vi "configuration UI.vi"() -> ()   [LabVIEW 2013, in "TEC editor node.lvclass"]
uses:
  TEC editor node.lvclass
  <vilib>/CEF_TreeControl/Node/NodeRef.ctl
  <vilib>/CEF_TreeControl/Node/NISE_CEF_Node.lvclass
  <vilib>/NI/AMC/Message Queue.ctl
  <vilib>/NI/AMC/Message.ctl
  <vilib>/NI/Tools/Keyed Array/KeyedArray.ctl
  <vilib>/CEF_TreeControl/Node/UserEventRef.ctl
  <vilib>/CEF_TreeControl/Controls/EventCluster.ctl
  <vilib>/NI/Tag Bus Data Framework/Configuration Editor/Classes/Engine Parent/Engine Parent Editor Node.lvclass
  <vilib>/NI/Tag Bus/tag/tag descriptor.lvclass
  <vilib>/NI/Tag Bus/tag/Data Type.ctl
  module/configuration/TEC configuration.lvclass
  <vilib>/NI/Module Execution Interface/Engine Configuration/engine configuration.lvclass
  <vilib>/NI/Tag Bus/tag/tag descriptor.lvclass/tag descriptor.ctl
  TEC editor node.lvclass/TEC editor node.ctl
  <vilib>/NI/Tag Bus Module Framework/channel/channel classification.ctl
  <vilib>/NI/Tag Bus Module Framework/root configuration/TBM configuration.lvclass/TBM configuration.ctl
  <vilib>/NI/Tag Bus/tag/write tag name.vi
  <vilib>/NI/Tag Bus/tag/write data type.vi
  <vilib>/NI/Tag Bus Module Framework/root configuration/create GUID.vi
  <vilib>/NI/Tag Bus Data Framework/Configuration Editor/Classes/Module editor node/module editor node.lvclass
  <vilib>/CEF_TreeControl/NISE_CEF_TreeControl.lvlib
  <vilib>/NI/Tag Bus Module Framework/channel/TBM channel.lvclass
  <vilib>/NI/Tag Bus Module Framework/root configuration/TBM configuration.lvclass
  <vilib>/NI/Tools/Keyed Array/Tools_KeyedArray.lvlib
  <vilib>/NI/AMC/AMC.lvlib
panel:
  in  "Tab Control":enum32{"Channel Mapping"}(tab)
  in  "Direction":T1(radio)
  in  "remove to":bool
  in  "add to":bool
  in  "remove from":bool
  in  "add from":bool
  in  "toCVTlist":i32(listbox)
  in  "fromCVTlist":i32(listbox)
  in  "avail tags":i32(listbox)=-1
  in  "user event":T2
  in  "main queue":T3
  in  "node ref":T4
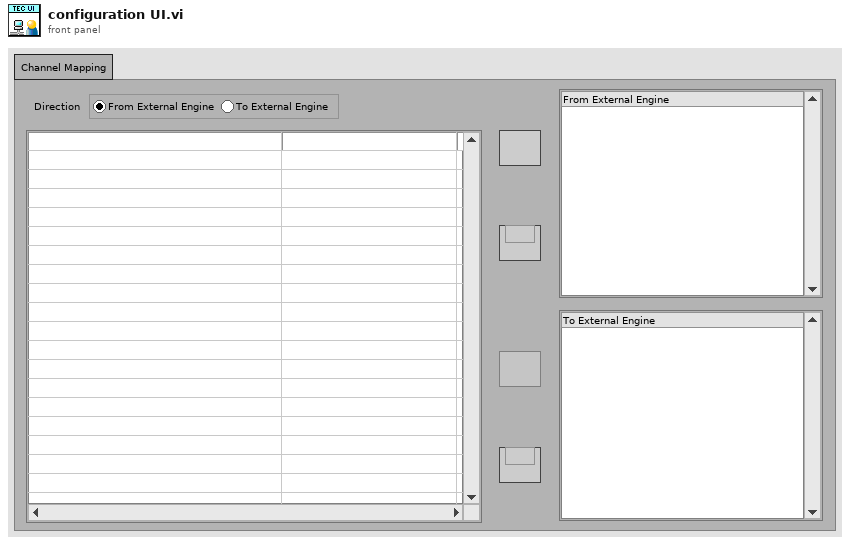
[diagram p1: front panel]
types:
  T1 = enum32{"From External Engine", "To External Engine"}
  T2 = typedef "NISE_CEF_Node.lvclass/UserEventRef.ctl" = refnum<user-event>
  T3 = typedef "AMC.lvlib/Message Queue.ctl" = refnum<queue>
  T4 = typedef "NISE_CEF_Node.lvclass/NodeRef.ctl" = refnum<data-value>
  T5 = typedef "NISE_CEF_TreeControl.lvlib/EventCluster.ctl" = cluster{"command":string, "data":string}
  T6 = typedef "tag bus.lvlib/tag descriptor.lvclass/Data Type.ctl" = enum16{"Double", "Single", "I64", "I32", "I16", "I8", "U64", "U32", "U16", "U8", "Boolean", "String", "Array of Double", "Array of Single", "Array of I64", "Array of I32", "Array of I16", "Array of I8", "Array of U64", "Array of U32", "Array of U16", "Array of U8", "Array of Boolean", "Array of String"}
  T7 = enum8{"Enabled", "Disabled", "Disabled and Grayed Out"}
  T8 = typedef "TBM channel.lvclass/channel classification.ctl" = enum16{"input data", "output data", "processing parameter", "processing result"}
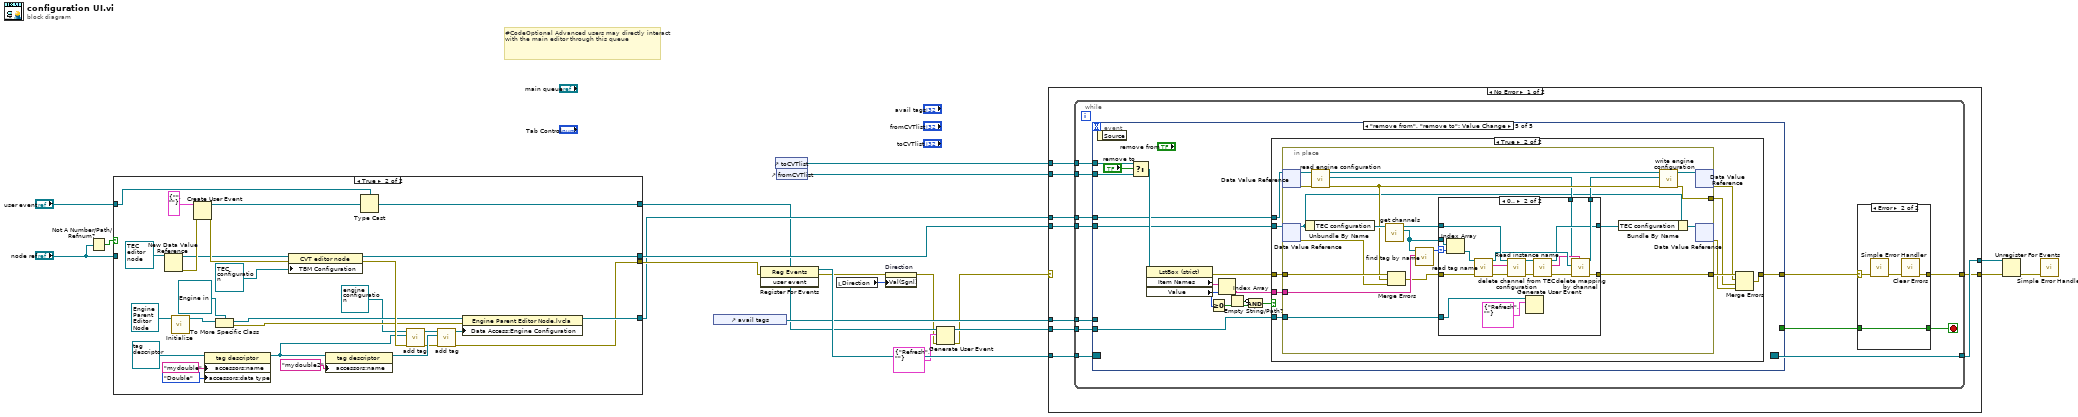
[diagram p0: block diagram]
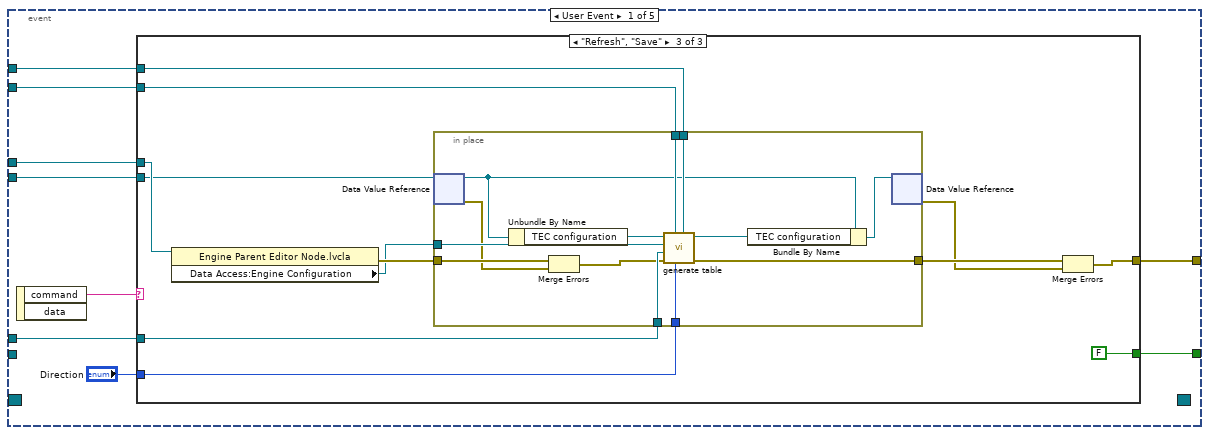
[diagram p3: hidden frame]
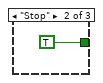
[diagram p5: hidden frame]
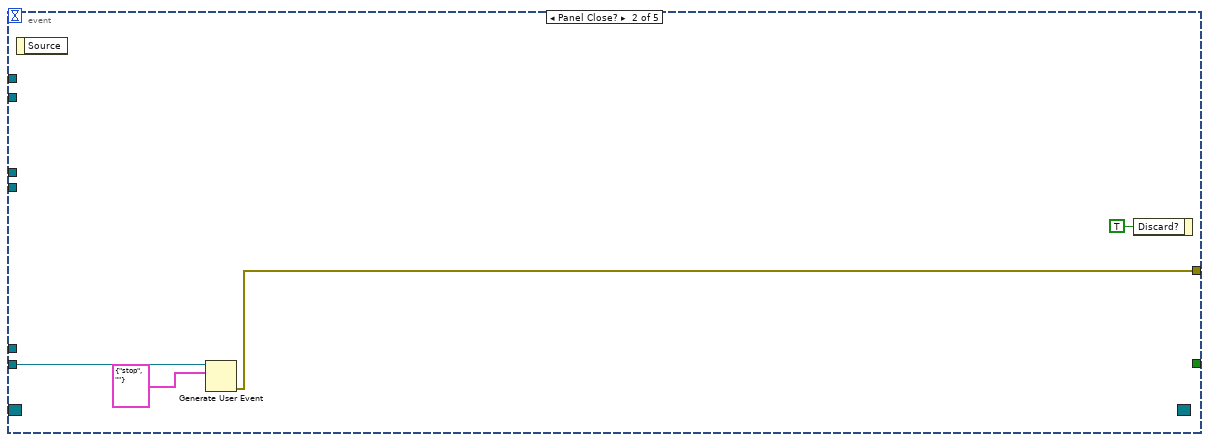
[diagram p6: hidden frame]
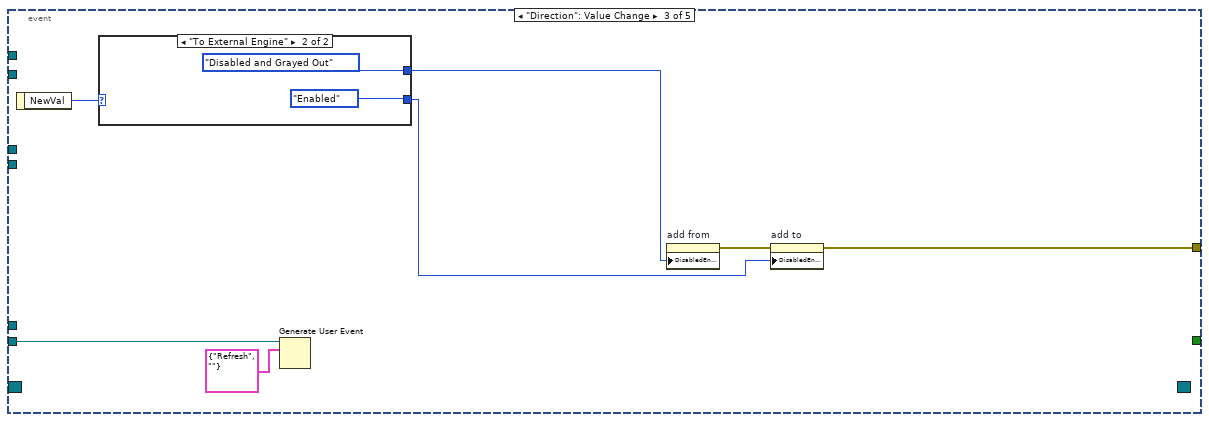
[diagram p7: hidden frame]
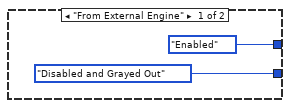
[diagram p8: hidden frame]
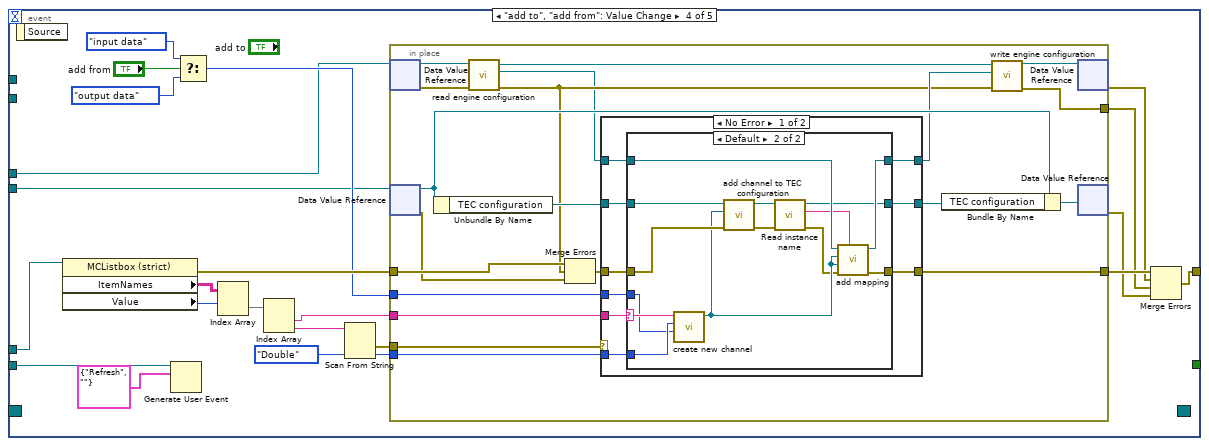
[diagram p9: hidden frame]
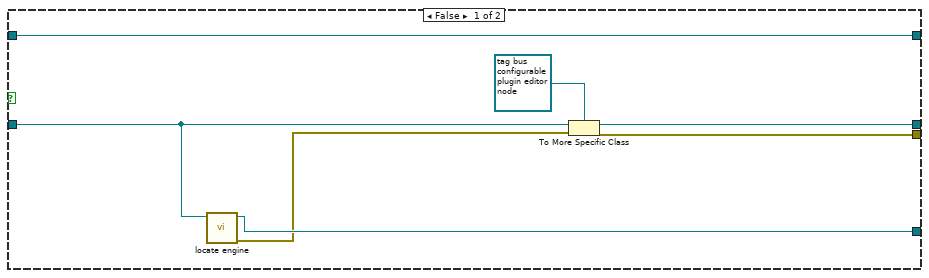
[diagram p15: hidden frame]
diagram:
  # "#CodeOptional Advanced users may directly interact with the main editor through this queue"
  n1 = Not A Number/Path/Refnum?(number/path/refnum="node ref") -> (NaN/Path/Refnum?=w17:bool)
  n2 = case shown="True" w17 {
    tunnel: "user event" -> [w27 w32]
    tunnel: [w27 w33] -> w3
    tunnel: "node ref" -> [w25 _]
    tunnel: [w24 w51] -> w14
    tunnel: [w23 w42] -> w13
    tunnel: [w22 w48] -> w11
    frame False {
      n3 = call <vilib>:"locate engine.vi"("component"=w25) -> ("error out"=w21:errorcluster, "engine"=w22:refnum<data-value>)  [unwired: 9 in]
      n4 = To More Specific Class(target class=refnum<data-value> refnum ("data value reference"), reference=w25, error in=w21) -> (specific class reference=w24:refnum<data-value>, error out=w23:errorcluster)
    }
    frame True {
      n5 = New Data Value Reference(data value=refnum<class "TEC editor node.lvclass"> refnum ("tag bus configurable plugin editor node")) -> (data value reference=w50:refnum<data-value>, error out=w53:errorcluster)  [unwired: 1 in]
      n6 = call-dynamic "Initialize.vi"("Engine in"=refnum<class "Engine Parent Editor Node.lvclass"> refnum) -> ("data value reference"=w37:T4)  [unwired: 8 in, 2 out]
      n7 = Create User Event(user event datatype=T5 {"command"="", "data"=""} ("event data"), error in=w53) -> (user event=w54:refnum<user-event>, error out=w52:errorcluster)
      n8 = property class="tag descriptor"(reference=refnum<class "tag descriptor.lvclass"> refnum ("tag descriptor"), "accessors:name"="mydouble" ("name"), "accessors:data type"=Data_Type."Double" ("data type")) -> (reference out=w40:refnum<class "tag descriptor.lvclass">)  [unwired: 1 in, 1 out]
      n9 = To More Specific Class(target class=refnum<data-value> refnum ("data value reference"), reference=w37) -> (specific class reference=w36:refnum<data-value>, error out=w34:errorcluster)  [unwired: 1 in]
      n10 = property class="CVT editor node"(reference=w50, error in=w52, "TBM Configuration"=refnum<class "TEC configuration.lvclass"> refnum ("CVT configuration")) -> (reference out=w51:refnum<data-value>, error out=w44:errorcluster)
      n11 = property class="tag descriptor"(reference=w40, "accessors:name"="mydouble2" ("name")) -> (reference out=w41:refnum<class "tag descriptor.lvclass">)  [unwired: 1 in, 1 out]
      n12 = Type Cast(type=w32, x=w54) -> (*(type *) &x=w33:T2)
      n13 = call <vilib>:"add tag.vi"("error in"=w44, "tag descriptor"=w40, "engine configuration in"=refnum<class "engine configuration.lvclass"> refnum) -> ("error out"=w31:errorcluster, "engine configuration out"=w30:refnum<class "engine configuration.lvclass">)  [unwired: 7 in]
      n14 = call <vilib>:"add tag.vi"("error in"=w31, "tag descriptor"=w41, "engine configuration in"=w30) -> ("error out"=w42:errorcluster, "engine configuration out"=w29:refnum<class "engine configuration.lvclass">)  [unwired: 7 in]
      n15 = property class="Engine Parent Editor Node.lvcla"(reference=w36, error in=w34, "Data Access:Engine Configuration"=w29) -> (reference out=w48:refnum<data-value>)  [unwired: 1 out]
    }
  }
  n16 = control-ref of="avail tags"() -> (w10:refnum<vi>)
  n17 = register-events(error in=w13, w3) -> (reference out=w20:refnum<event-registration>, error out=w7:errorcluster)  [unwired: 1 in]
  n18 = control-ref of="toCVTlist"() -> (w9:refnum<vi>)
  n19 = control-ref of="fromCVTlist"() -> (w8:refnum<vi>)
  n20 = local read "Direction"() -> (w6:T1)
  n21 = property on="Direction" class="RadioBtnsControl (strict)"(error in=w7, "Val(Sgnl)"=w6) -> (error out=w2:errorcluster)  [unwired: 1 in, 1 out]
  n22 = Generate User Event(user event=w3, event data cluster=T5 {"command"="Refresh", "data"=""} ("event data"), error in=w2) -> (user event out=w4:T2, error out=w1:errorcluster)  [unwired: 1 in]
  n23 = case shown="No Error" w1 {
    selector: w1 -> [_ w274]
    tunnel: w20 -> [w64 w273]
    tunnel: [w63 w273] -> w19
    tunnel: [w62 w274] -> w18
    tunnel: w14 -> [w61 _]
    tunnel: w11 -> [w60 _]
    tunnel: w10 -> [w59 _]
    tunnel: w9 -> [w58 _]
    tunnel: w8 -> [w57 _]
    tunnel: w4 -> [w56 _]
    frame No Error {
      n24 = while {
        tunnel: w64 -> [w76]
        tunnel: [w75] -> w63
        tunnel: w61 -> [w70]
        tunnel: w60 -> [w69]
        tunnel: w56 -> [w68]
        tunnel: w59 -> [w67]
        tunnel: w58 -> [w66]
        tunnel: w57 -> [w65]
        tunnel: [w71] -> w62
        stop <- w73 stop-if-true
        n25 = event shown="[4] \"remove from\", \"remove to\": Value Change" {
          selector: w76 -> [_ _ _ _ _]
          dyn-events: [_ _ _ _ _] -> w75
          timeout: _ -> [_ _ _ _ _]
          tunnel: [w91 _ _ _ _] -> w72
          tunnel: [w89 w118 w125 w138 w209] -> w74
          tunnel: w70 -> [w88 _ _ w134 w206]
          tunnel: w69 -> [w87 _ _ w135 w205]
          tunnel: w68 -> [_ w119 w127 w154 w208]
          tunnel: w67 -> [w86 _ _ w148 _]
          tunnel: w66 -> [w85 _ _ _ w218]
          tunnel: w65 -> [w84 _ _ _ w219]
          event User Event {
            n26 = event-data() -> ("command"=w90:string)  [unwired: 1 in, 1 out]
            n27 = case shown="\"Refresh\", \"Save\"" w90 {
              tunnel: [_ TRUE FALSE] -> w91
              tunnel: [_ _ w94] -> w89
              tunnel: w88 -> [_ _ w95]
              tunnel: w87 -> [_ _ w97]
              tunnel: w86 -> [_ _ w102]
              tunnel: w85 -> [_ _ w101]
              tunnel: w84 -> [_ _ w100]
              tunnel: "Direction" -> [_ _ w99]
              frame Default {
              }
              frame "Stop" {
              }
              frame "Refresh", "Save" {
                n28 = property class="Engine Parent Editor Node.lvcla"(reference=w97) -> (error out=w98:errorcluster, "Data Access:Engine Configuration"=w96:refnum<class "engine configuration.lvclass">)  [unwired: 1 in, 1 out]
                n29 = in-place {
                  in-place-border: [w117] -> w103
                  in-place-border: w102 -> [w116]
                  in-place-border: w101 -> [w115]
                  in-place-border: w100 -> [w114]
                  in-place-border: w99 -> [w113]
                  in-place-border: w98 -> [w112]
                  in-place-border: w96 -> [w111]
                  n30 = in-place-dvr #1(w95) -> (w107:refnum<class "TEC editor node.lvclass">, w109:errorcluster)
                  n31 = Unbundle By Name(w107) -> ("TEC configuration"=w108:refnum<class "TEC configuration.lvclass">)
                  n32 = Merge Errors(w112, w109) -> (w110:errorcluster)
                  n33 = call "generate table.vi"("to TEC"=w115, "Direction"=w113, "from TEC"=w114, "error in"=w110, "avail tags"=w116, "engine configuration in"=w111, "TEC in"=w108) -> ("error out"=w117:errorcluster, "TEC out"=w105:refnum<class "TEC configuration.lvclass">)  [unwired: 3 in]
                  n34 = Bundle By Name(cluster=w107, "TEC configuration"=w105) -> (w106:refnum<class "TEC editor node.lvclass">)
                  n35 = in-place-dvr #1(w106) -> (w93:errorcluster)  [unwired: 1 out]
                }
                n36 = Merge Errors(w103, w93) -> (w94:errorcluster)
              }
            }
          }
          event Panel Close? {
            n37 = event-data() -> ()  [unwired: 1 in, 1 out]
            n38 = Generate User Event(user event=w119, event data cluster=T5 {"command"="stop", "data"=""} ("event data")) -> (error out=w118:errorcluster)  [unwired: 2 in, 1 out]
            n39 = event-data("Discard?"=TRUE) -> ()  [unwired: 1 in, 1 out]
          }
          event "Direction": Value Change {
            n40 = event-data() -> ("NewVal"=w124:T1)  [unwired: 1 in]
            n41 = case shown="\"To External Engine\"" w124 {
              tunnel: [T7."Enabled" ("Disabled") T7."Disabled and Grayed Out" ("Disabled")] -> w123
              tunnel: [T7."Disabled and Grayed Out" ("Disabled") T7."Enabled" ("Disabled")] -> w122
              frame "From External Engine" {
              }
              frame "To External Engine" {
              }
            }
            n42 = Generate User Event(user event=w127, event data cluster=T5 {"command"="Refresh", "data"=""} ("event data")) -> ()  [unwired: 2 in, 2 out]
            n43 = property on="add from" class="Bool"("DisabledEnum"=w123) -> (error out=w126:errorcluster)  [unwired: 2 in, 1 out]
            n44 = property on="add to" class="Bool"(error in=w126, "DisabledEnum"=w122) -> (error out=w125:errorcluster)  [unwired: 1 in, 1 out]
          }
          event "add to", "add from": Value Change {
            n45 = event-data() -> ()  [unwired: 1 in, 1 out]
            n46 = property class="MCListbox (strict)"(reference=w148) -> (error out=w149:errorcluster, "ItemNames"=w147:string[][], "Value"=w146:i32)  [unwired: 1 in, 1 out]
            n47 = Generate User Event(user event=w154, event data cluster=T5 {"command"="Refresh", "data"=""} ("event data")) -> ()  [unwired: 2 in, 2 out]
            n48 = Select(t=channel_classification."input data" ("channel classification"), s="add from", f=channel_classification."output data" ("channel classification")) -> (s? t:f=w139:T8)
            n49 = Index Array(array=w147, index (row)=w146) -> (element=w143:string[])  [unwired: 1 in]
            n50 = Index Array(array=w143) -> (element #1=w142:string, element #2=w145:string)  [unwired: 2 in]
            n51 = Scan From String(input string=w145, default 1=Data_Type."Double" ("data type")) -> (error out=w141:errorcluster, output 1=w140:T6)  [unwired: 3 in, 2 out]
            n52 = in-place {
              in-place-border: [w175] -> w155
              in-place-border: w149 -> [w174]
              in-place-border: w142 -> [w173]
              in-place-border: w141 -> [w172]
              in-place-border: w140 -> [w171]
              in-place-border: w139 -> [w170]
              in-place-border: [w160] -> w133
              n53 = in-place-dvr #2(w135) -> (w163:refnum<class "Engine Parent Editor Node.lvclass">, w158:errorcluster)
              n54 = in-place-dvr #3(w134) -> (w166:refnum<class "TEC editor node.lvclass">, w164:errorcluster)
              n55 = Unbundle By Name(w166) -> ("TEC configuration"=w168:refnum<class "TEC configuration.lvclass">)
              n56 = call <vilib>:"read engine configuration.vi"("error in"=w158, "Engine Parent Editor Node in"=w163) -> ("error out"=w157:errorcluster, "engine configuration"=w156:refnum<class "engine configuration.lvclass">, "Engine Parent Editor Node out"=w159:refnum<class "Engine Parent Editor Node.lvclass">)  [unwired: 7 in]
              n57 = Merge Errors(w174, w157, w164) -> (w169:errorcluster)
              n58 = case shown="No Error" w172 {
                tunnel: [w184 w202] -> w175
                tunnel: [w183 w204] -> w161
                tunnel: [w182 w203] -> w167
                tunnel: w168 -> [w181 w203]
                tunnel: w156 -> [w180 w204]
                tunnel: w169 -> [w179 w202]
                tunnel: w173 -> [w178 _]
                tunnel: w171 -> [w177 _]
                tunnel: w170 -> [w176 _]
                frame No Error {
                  n59 = case shown="Default" w178 {
                    selector: w178 -> [_ w195]
                    tunnel: [w187 w201] -> w184
                    tunnel: w179 -> [w187 w197]
                    tunnel: w180 -> [w185 w200]
                    tunnel: [w186 w189] -> w182
                    tunnel: w181 -> [w186 w198]
                    tunnel: [w185 w199] -> w183
                    tunnel: w177 -> [_ w194]
                    tunnel: w176 -> [_ w193]
                    frame "" {
                    }
                    frame Default {
                      n60 = call <vilib>:"create new channel.vi"("channel classification"=w193, "data type"=w194, "channel name"=w195) -> ("channel"=w192:refnum<class "TBM channel.lvclass">)  [unwired: 8 in]
                      n61 = call "add channel to TEC configuration.vi"("error in"=w197, "channel"=w192, "TEC configuration in"=w198) -> ("error out"=w196:errorcluster, "TEC configuration out"=w190:refnum<class "TEC configuration.lvclass">)  [unwired: 7 in]
                      n62 = call <vilib>:"Read instance name.vi"("error in"=w196, "configuration in"=w190) -> ("error out"=w191:errorcluster, "instance id"=w188:string, "configuration out"=w189:refnum<class "TEC configuration.lvclass">)  [unwired: 7 in]
                      n63 = call <vilib>:"add mapping.vi"("owner ID"=w188, "error in"=w191, "channel"=w192, "tag descriptor"=w192, "engine configuration"=w200) -> ("error out"=w201:errorcluster, "engine configuration out"=w199:refnum<class "engine configuration.lvclass">)  [unwired: 5 in]
                    }
                  }
                }
                frame Error {
                }
              }
              n64 = Bundle By Name(cluster=w166, "TEC configuration"=w167) -> (w165:refnum<class "TEC editor node.lvclass">)
              n65 = call <vilib>:"write engine configuration.vi"("error in"=w157, "engine configuration"=w161, "Engine Parent Editor Node in"=w159) -> ("error out"=w160:errorcluster, "Engine Parent Editor Node out"=w162:refnum<class "Engine Parent Editor Node.lvclass">)  [unwired: 7 in]
              n66 = in-place-dvr #2(w162) -> (w137:errorcluster)  [unwired: 1 out]
              n67 = in-place-dvr #3(w165) -> (w136:errorcluster)  [unwired: 1 out]
            }
            n68 = Merge Errors(w155, w137, w133, w136) -> (w138:errorcluster)
          }
          event "remove from", "remove to": Value Change {
            n69 = event-data() -> ()  [unwired: 1 in, 1 out]
            n70 = Select(t=w218, s="remove to", f=w219) -> (s? t:f=w216:refnum<vi>)
            n71 = property class="LstBox (strict)"(reference=w216) -> (error out=w210:errorcluster, "Item Names"=w215:string[], "Value"=w214:i32)  [unwired: 1 in, 1 out]
            n72 = Greater Or Equal To 0?(x=w214) -> (x >= 0?=w212:bool)
            n73 = Index Array(array=w215, index=w214) -> (element=w207:string)
            n74 = Empty String/Path?(string/path=w207) -> (empty?=w213:bool)
            n75 = Compound Arithmetic op=AND(invert w213, w212) -> (w211:bool)
            n76 = case shown="True" w211 {
              tunnel: w210 -> [w220 w227]
              tunnel: [w220 w226] -> w209
              tunnel: w208 -> [_ w230]
              tunnel: w207 -> [_ w229]
              tunnel: w206 -> [_ w225]
              tunnel: w205 -> [_ w224]
              frame False {
              }
              frame True {
                n77 = in-place {
                  in-place-border: w230 -> [w251]
                  in-place-border: w229 -> [w250]
                  in-place-border: [w247] -> w228
                  in-place-border: w227 -> [w246]
                  in-place-border: [w240] -> w221
                  n78 = in-place-dvr #4(w224) -> (w243:refnum<class "Engine Parent Editor Node.lvclass">, w238:errorcluster)
                  n79 = in-place-dvr #5(w225) -> (w233:refnum<class "TEC editor node.lvclass">, w237:errorcluster)
                  n80 = Unbundle By Name(w233) -> ("TEC configuration"=w239:refnum<class "TEC configuration.lvclass">)
                  n81 = call <vilib>:"read engine configuration.vi"("error in"=w238, "Engine Parent Editor Node in"=w243) -> ("error out"=w236:errorcluster, "engine configuration"=w235:refnum<class "engine configuration.lvclass">, "Engine Parent Editor Node out"=w242:refnum<class "Engine Parent Editor Node.lvclass">)  [unwired: 7 in]
                  n82 = call-dynamic "get channels.vi"("TEC configuration in"=w239) -> ("channels"=w245:refnum<class "TBM channel.lvclass">[], "TEC configuration out"=w248:refnum<class "TEC configuration.lvclass">)  [unwired: 9 in]
                  n83 = Merge Errors(w246, w236, w237) -> (w244:errorcluster)
                  n84 = call <vilib>:"find tag by name.vi"("name"=w250, "tags in"=w245) -> ("index"=w249:i32)  [unwired: 9 in]
                  n85 = case shown="0.." w249 {
                    selector: w249 -> [_ w270]
                    tunnel: w251 -> [_ w271]
                    tunnel: w248 -> [w254 w268]
                    tunnel: [w254 w257] -> w231
                    tunnel: [w253 w264] -> w247
                    tunnel: w244 -> [w253 w267]
                    tunnel: [w252 w265] -> w234
                    tunnel: w245 -> [_ w269]
                    tunnel: w235 -> [w252 w255]
                    frame ..-1 {
                    }
                    frame 0.. {
                      n86 = Index Array(array=w269, index=w270) -> (element=w262:refnum<class "TBM channel.lvclass">)
                      n87 = call <vilib>:"read tag name.vi"("error in"=w267, "system tag in"=w262) -> ("error out"=w263:errorcluster, "name"=w260:string, "system tag out"=w261:refnum<class "TBM channel.lvclass">)  [unwired: 7 in]
                      n88 = call "delete channel from TEC configuration.vi"("error in"=w263, "channel to delete"=w260, "TEC configuration in"=w268) -> ("error out"=w266:errorcluster, "TEC configuration out"=w258:refnum<class "TEC configuration.lvclass">)  [unwired: 7 in]
                      n89 = Generate User Event(user event=w271, event data cluster=T5 {"command"="Refresh", "data"=""} ("event data")) -> ()  [unwired: 2 in, 2 out]
                      n90 = call <vilib>:"Read instance name.vi"("error in"=w266, "configuration in"=w258) -> ("error out"=w259:errorcluster, "instance id"=w256:string, "configuration out"=w257:refnum<class "TEC configuration.lvclass">)  [unwired: 7 in]
                      n91 = call <vilib>:"delete mapping by channel.vi"("owner ID"=w256, "error in"=w259, "channel"=w261, "engine configuration in"=w255) -> ("error out"=w264:errorcluster, "engine configuration out"=w265:refnum<class "engine configuration.lvclass">)  [unwired: 6 in]
                    }
                  }
                  n92 = Bundle By Name(cluster=w233, "TEC configuration"=w231) -> (w232:refnum<class "TEC editor node.lvclass">)
                  n93 = call <vilib>:"write engine configuration.vi"("error in"=w236, "engine configuration"=w234, "Engine Parent Editor Node in"=w242) -> ("error out"=w240:errorcluster, "Engine Parent Editor Node out"=w241:refnum<class "Engine Parent Editor Node.lvclass">)  [unwired: 7 in]
                  n94 = in-place-dvr #4(w241) -> (w223:errorcluster)  [unwired: 1 out]
                  n95 = in-place-dvr #5(w232) -> (w222:errorcluster)  [unwired: 1 out]
                }
                n96 = Merge Errors(w228, w223, w221, w222) -> (w226:errorcluster)
              }
            }
          }
        }
        n97 = case shown="Error" w74 {
          selector: w74 -> [w77 w81]
          tunnel: [w78 w82] -> w73
          tunnel: w72 -> [w78 w82]
          tunnel: [w77 w79] -> w71
          frame No Error {
          }
          frame Error {
            n98 = call <vilib>:"Simple Error Handler.vi"("error in (no error)"=w81) -> ("error out"=w80:errorcluster)  [unwired: 4 in, 4 out]
            n99 = call <vilib>:"Clear Errors.vi"("error in (no error)"=w80) -> ("error out"=w79:errorcluster)  [unwired: 6 in]
          }
        }
      }
    }
    frame Error {
    }
  }
  n100 = Unregister For Events(event registration refnum=w19, error in=w18) -> (error out=w12:errorcluster)
  n101 = call <vilib>:"Simple Error Handler.vi"("error in (no error)"=w12) -> ()  [unwired: 4 in, 5 out]
